vi "initialize.vi"(8 "error in (no error)":errorcluster, 11 "lv-builder in":refnum<class "lv-builder.lvclass">) -> (0 "error out":errorcluster, 3 "lv-builder out":refnum<class "lv-builder.lvclass">)   [LabVIEW 2015, in "lv-builder.lvlib" / "lv-builder.lvclass"]
uses:
  lv-builder.lvclass
  public/_controls/configuration.ctl
  <userlib>/antonio-alexander/lv-bin/public/api/v1/advanced/add_data_path_single.vi
  lv-builder.lvlib
  <userlib>/antonio-alexander/lv-bin-git/public/api/v1/v1.lvlib
  <userlib>/antonio-alexander/lv-bin/public/api/v1/v1.lvlib
  <userlib>/antonio-alexander/lv-bin-7zip/lv-bin-7zip.lvlib
  <userlib>/antonio-alexander/lv-bin-git/lv-bin-git.lvlib
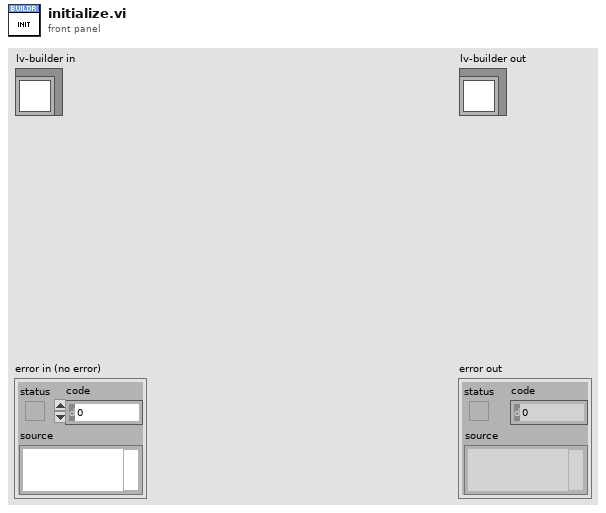
[diagram p1: front panel]
types:
  T1 = typedef "lv-builder.lvlib/configuration.ctl" = cluster{"project_file":string, "lvlibp_directory":string, "zip_directory":string, "lvlib_directory":string, "update_version_vi":string, "installer_post_file":string, "lvlib_post_action":u16, "installer_post_action":u16, "application_post_action":u16, "zip_post_action":u16}
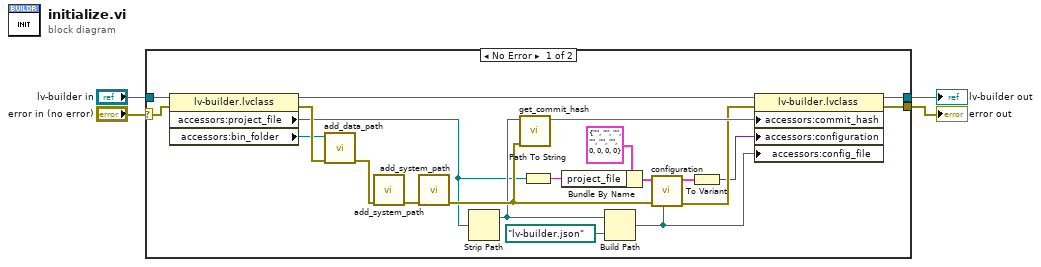
[diagram p0: block diagram]
diagram:
  n1 = case shown="No Error" "error in (no error)" {
    selector: "error in (no error)" -> [w7 w27]
    tunnel: [w8 w27] -> w3
    tunnel: [w10 w26] -> w1
    tunnel: "lv-builder in" -> [w24 w26]
    frame No Error {
      n2 = property class="lv-builder.lvclass"(reference=w24, error in=w7) -> (reference out=w11:refnum<class "lv-builder.lvclass">, error out=w25:errorcluster, "accessors:project_file"=w13:path, "accessors:bin_folder"=w12:path)
      n3 = call-poly <userlib>:"add_data_path.vi"("error in (no error)"=w25, "path_to_add"=w12) -> ("error out"=w18:errorcluster)  [unwired: 9 in]
      n4 = call <userlib>:"add_system_path.vi"("error in (no error)"=w18) -> ("error out"=w17:errorcluster)  [unwired: 10 in]
      n5 = call <userlib>:"add_system_path.vi"("error in (no error)"=w17) -> ("error out"=w23:errorcluster)  [unwired: 10 in]
      n6 = Strip Path(path=w13) -> (stripped path=w21:path)  [unwired: 1 out]
      n7 = call <userlib>:"get_commit_hash.vi"("error in (no error)"=w23, "path"=w21) -> ("commit_hash"=w19:string)  [unwired: 8 in, 1 out]
      n8 = Path To String(path=w13) -> (string=w14:string)
      n9 = Bundle By Name(cluster=T1 {"project_file"="", "lvlibp_directory"="", "zip_directory"="", "lvlib_directory"="", "update_version_vi"="", "installer_post_file"="", "lvlib_post_action"=0, "installer_post_action"=0, "application_post_action"=0, "zip_post_action"=0} ("config in"), "project_file"=w14) -> (w15:T1)
      n10 = Build Path(base path=w21, name or relative path=path "lv-builder.json" ("stripped path")) -> (appended path=w5:path)
      n11 = call "configuration.vi"("config_file"=w5, "error in (no error)"=w23, "config in"=w15) -> ("error out"=w9:errorcluster, "config out"=w20:T1)  [unwired: 7 in]
      n12 = To Variant(anything=w20) -> (Variant=w6:variant)
      n13 = property class="lv-builder.lvclass"(reference=w11, error in=w9, "accessors:commit_hash"=w19, "accessors:configuration"=w6, "accessors:config_file"=w5) -> (reference out=w10:refnum<class "lv-builder.lvclass">, error out=w8:errorcluster)
    }
    frame Error {
    }
  }
  "error out" <- w3
  "lv-builder out" <- w1
